vi "TestEventRx.vi"() -> ()   [LabVIEW 2017]
uses:
  zmq_utilities/TTLReceive.vi
  <vilib>/addons/zeromq/zmq_recv_multi.vi
panel:
  out "error out":errorcluster
  out "crossing time":i64
  out "learning rate":dbl
  out "crossing level":sgl
  out "event time":i64
  in  "channel":u16=1 min=1 max=8
  out "threshold":sgl
  out "rising?":bool
  in  "Stop Button":bool
  in  "port":u16=5557
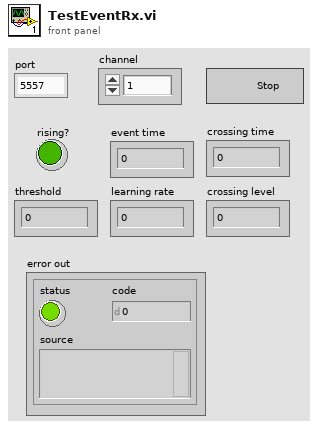
[diagram p1: front panel]
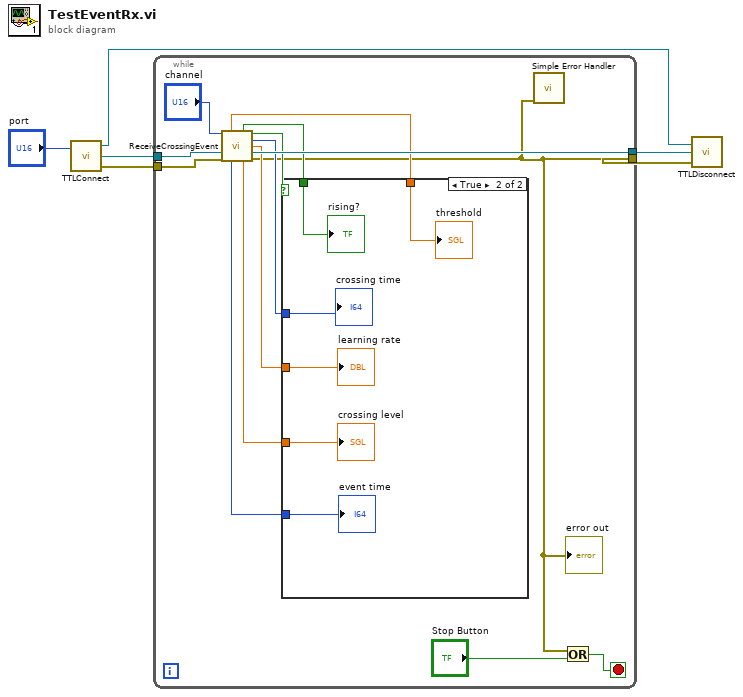
[diagram p0: block diagram]
diagram:
  n1 = call "TTLConnect.vi"("port"="port") -> ("context out"=w5:refnum<class "zmq_context.lvclass">, "socket out"=w4:refnum<class "zmq_socket.lvclass">, "error out"=w2:errorcluster)  [unwired: 1 in]
  n2 = while {
    tunnel: w4 -> [w20]
    tunnel: [w19] -> w3
    tunnel: w2 -> [w18]
    tunnel: [w9] -> w1
    stop <- w7 stop-if-true
    n3 = call "ReceiveCrossingEvent.vi"("channel"="channel", "socket in"=w20, "error in"=w18) -> ("threshold"=w15:sgl, "rising?"=w16:bool, "new crossing"=w17:bool, "crossing time"=w10:i64, "learning rate"=w11:dbl, "socket out"=w19:refnum<class "zmq_socket.lvclass">, "event time"=w13:i64, "crossing level"=w12:sgl, "error out"=w9:errorcluster)  [unwired: 4 in]
    "error out" <- w9
    n4 = case shown="True" w17 {
      tunnel: w16 -> [_ w26]
      tunnel: w15 -> [_ w25]
      tunnel: w13 -> [_ w24]
      tunnel: w12 -> [_ w23]
      tunnel: w11 -> [_ w22]
      tunnel: w10 -> [_ w21]
      frame False {
      }
      frame True {
        "rising?" <- w26
        "threshold" <- w25
        "event time" <- w24
        "crossing level" <- w23
        "learning rate" <- w22
        "crossing time" <- w21
      }
    }
    n5 = call <vilib>:"Simple Error Handler.vi"("error in (no error)"=w9) -> ()  [unwired: 4 in, 5 out]
    n6 = Or(x=w9, y="Stop Button") -> (x .or. y?=w7:bool)
  }
  n7 = call "TTLDisconnect.vi"("error in"=w1, "socket in"=w3, "context in"=w5) -> ()  [unwired: 1 in, 1 out]
